vi "筛选XML解决方案.vi"(8 "error in (no error)":errorcluster caption="错误输入（无错误）", 11 "筛选输入":cluster{"platform_alarm_code":string}={"platform_alarm_code"="010002013"}) -> (0 "error out":errorcluster caption="错误输出", 3 "data":T1(array[cluster]))   [LabVIEW 2016, in "Alarm interface.lvlib"]
uses:
  Alarm interface.lvlib
  <vilib>/xml/Load XML File.vi
  <vilib>/xml/Close Reference(Node).vi
  <vilib>/xml/NI_XML.lvlib
  <resource>/objmgr/DOMUserDefRef.rc
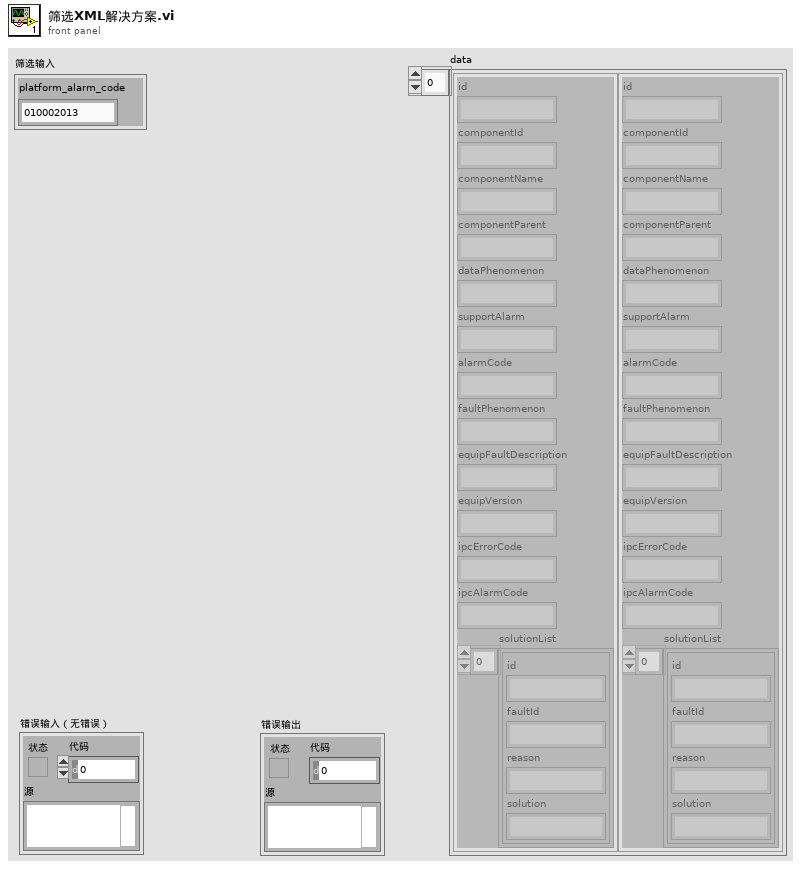
[diagram p1: front panel]
types:
  T1 = cluster{"id":string, "componentId":string, "componentName":string, "componentParent":string, "dataPhenomenon":string, "supportAlarm":string, "alarmCode":string, "faultPhenomenon":string, "equipFaultDescription":string, "equipVersion":string, "ipcErrorCode":string, "ipcAlarmCode":string, "solutionList":cluster{"id":string, "faultId":string, "reason":string, "solution":string}[]}[]
  T2 = cluster{"node text":string, "node text":string, "node text":string, "node text":string}
  T3 = cluster{"id":string, "componentId":string, "componentName":string, "componentParent":string, "dataPhenomenon":string, "supportAlarm":string, "alarmCode":string, "faultPhenomenon":string, "equipFaultDescription":string, "equipVersion":string, "ipcErrorCode":string, "ipcAlarmCode":string, "solutionList":cluster{"id":string, "faultId":string, "reason":string, "solution":string}[]}
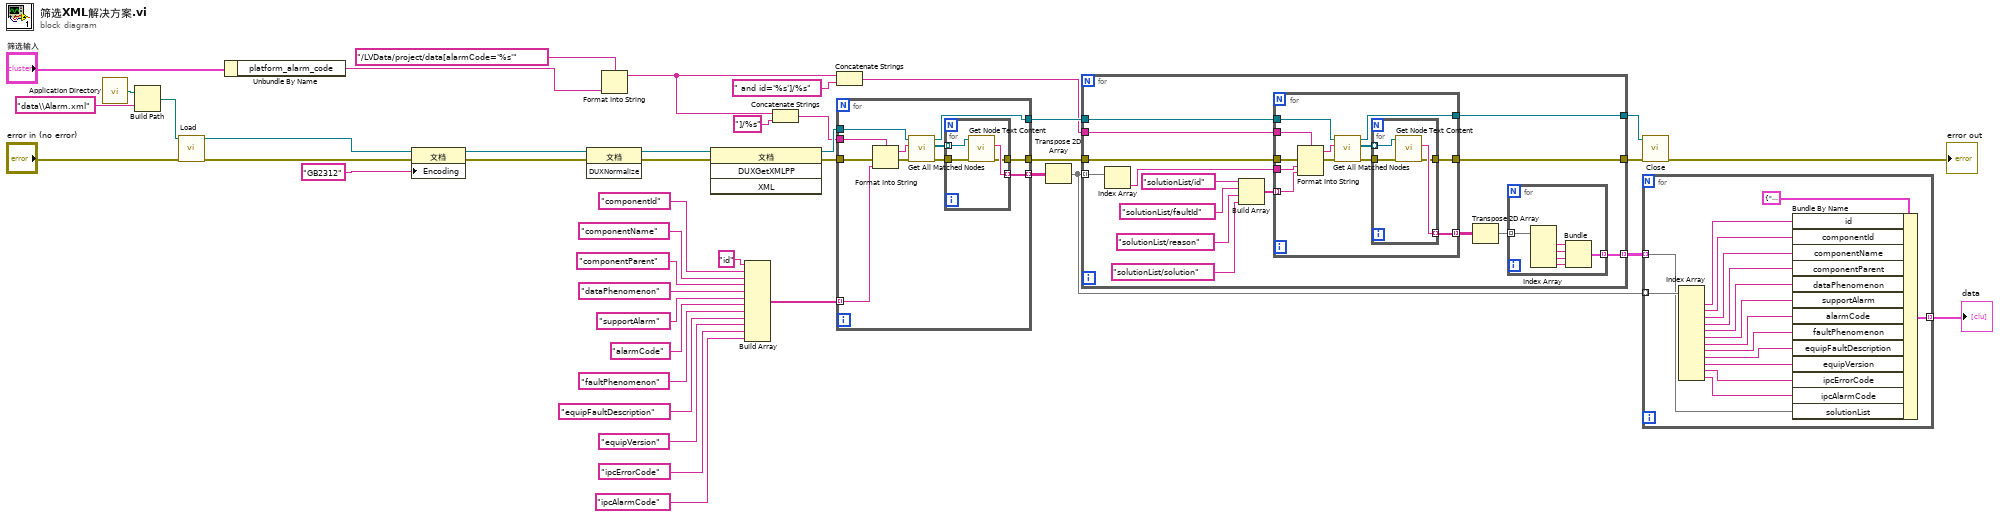
[diagram p0: block diagram]
diagram:
  n1 = call <vilib>:"Application Directory.vi"() -> ("Application Directory"=w4:path)
  n2 = Build Path(base path=w4, name or relative path="data\\Alarm.xml" ("字符串")) -> (appended path=w2:path)
  n3 = call-poly <vilib>:"Load.vi"("path to XML document"=w2, "error in (no error)"="error in (no error)") -> ("DOM document out"=w40:refnum<k20>, "error out"=w39:errorcluster)  [unwired: 11 in, 1 out]
  n4 = Unbundle By Name("筛选输入") -> ("platform_alarm_code"=w5:string)
  n5 = property on="属性节点" class="文档"(reference=w40, error in=w39, "Encoding"="GB2312" ("文档编码")) -> (reference out=w42:refnum<k20>, error out=w41:errorcluster)
  n6 = invoke on="调用节点" class="文档" method="DUXNormalize"(reference=w42, error in=w41) -> (reference out=w38:refnum<k20>, error out=w37:errorcluster)  [unwired: 1 in, 1 out]
  n7 = Format Into String(format string="/LVData/project/data[alarmCode='%s'" ("字符串"), w5) -> (resulting string=w14:string)  [unwired: 2 in, 1 out]
  n8 = invoke on="调用节点" class="文档" method="DUXGetXMLPP"(reference=w38, error in=w37) -> (reference out=w24:refnum<k20>, error out=w9:errorcluster)  [unwired: 2 in, 2 out]
  n9 = Build Array("id", "componentId", "componentName", "componentParent", "dataPhenomenon", "supportAlarm", "alarmCode", "faultPhenomenon", "equipFaultDescription", "equipVersion", "ipcErrorCode", "ipcAlarmCode") -> (w23:string[])
  n10 = Concatenate Strings(w14, "]/%s" ("字符串")) -> (w15:string)
  n11 = Concatenate Strings(w14, " and id='%s']/%s" ("字符串")) -> (w12:string)
  n12 = for {
    tunnel: w24 -> [w54]
    tunnel: w15 -> [w53]
    tunnel: w23 -> [w51] mode=indexing
    tunnel: [w49] -> w22 mode=indexing
    tunnel: [w48] -> w21
    tunnel: [w45] -> w10
    tunnel: w9 -> [w44]
    n13 = Format Into String(format string=w53, error in=w44, w51) -> (resulting string=w52:string, error out=w47:errorcluster)  [unwired: 1 in]
    n14 = call <vilib>:"Get All Matched Nodes.vi"("error in (no error)"=w47, "XPath expression"=w52, "node in"=w54) -> ("error out"=w46:errorcluster, "node result array"=w50:refnum<k20>[], "node out"=w48:refnum<k20>)  [unwired: 6 in]
    n15 = for {
      tunnel: w50 -> [w58] mode=indexing
      tunnel: [w57] -> w49 mode=indexing
      tunnel: w46 -> [w56]
      tunnel: [w55] -> w45
      n16 = call <vilib>:"Get Node Text Content.vi"("error in (no error)"=w56, "node in"=w58) -> ("error out"=w55:errorcluster, "node text"=w57:string)  [unwired: 7 in, 1 out]
    }
  }
  n17 = Transpose 2D Array(2D array=w22) -> (transposed array=w18:string[][])
  n18 = for {
    tunnel: w18 -> [w73] mode=indexing
    tunnel: w12 -> [w72]
    tunnel: w21 -> [w70]
    tunnel: [w63] -> w20
    tunnel: [w61] -> w19 mode=indexing
    tunnel: w10 -> [w60]
    tunnel: [w59] -> w8
    n19 = Index Array(array=w73) -> (element=w71:string)  [unwired: 1 in]
    n20 = Build Array("solutionList/id" ("XPath expression"), "solutionList/faultId" ("XPath expression"), "solutionList/reason" ("XPath expression"), "solutionList/solution" ("XPath expression")) -> (w65:string[])
    n21 = for {
      tunnel: w72 -> [w91]
      tunnel: w71 -> [w90]
      tunnel: w65 -> [w89] mode=indexing
      tunnel: w70 -> [w87]
      tunnel: [w85] -> w64 mode=indexing
      tunnel: [w84] -> w63
      tunnel: w60 -> [w83]
      tunnel: [w80] -> w59
      n22 = Format Into String(format string=w91, error in=w83, w90, w89) -> (resulting string=w86:string, error out=w82:errorcluster)  [unwired: 1 in]
      n23 = call <vilib>:"Get All Matched Nodes.vi"("error in (no error)"=w82, "XPath expression"=w86, "node in"=w87) -> ("error out"=w81:errorcluster, "node result array"=w88:refnum<k20>[], "node out"=w84:refnum<k20>)  [unwired: 6 in]
      n24 = for {
        tunnel: w88 -> [w95] mode=indexing
        tunnel: [w94] -> w85 mode=indexing
        tunnel: w81 -> [w93]
        tunnel: [w92] -> w80
        n25 = call <vilib>:"Get Node Text Content.vi"("error in (no error)"=w93, "node in"=w95) -> ("error out"=w92:errorcluster, "node text"=w94:string)  [unwired: 7 in, 1 out]
      }
    }
    n26 = Transpose 2D Array(2D array=w64) -> (transposed array=w62:string[][])
    n27 = for {
      tunnel: w62 -> [w79] mode=indexing
      tunnel: [w74] -> w61 mode=indexing
      n28 = Index Array(array=w79) -> (element #1=w78:string, element #2=w77:string, element #3=w76:string, element #4=w75:string)  [unwired: 4 in]
      n29 = Bundle("node text"=w78, "node text"=w77, "node text"=w76, "node text"=w75) -> (w74:T2)  [unwired: 1 in]
    }
  }
  n30 = call-poly <vilib>:"Close.vi"("error in (no error)"=w8, "node"=w20) -> ("error out"=→"error out":errorcluster)  [unwired: 7 out]
  n31 = for {
    tunnel: w18 -> [w97] mode=indexing
    tunnel: [w98] -> w17 mode=indexing
    tunnel: w19 -> [w96] mode=indexing
    n32 = Index Array(array=w97) -> (element #1=w110:string, element #2=w109:string, element #3=w108:string, element #4=w107:string, element #5=w106:string, element #6=w105:string, element #7=w104:string, element #8=w103:string, element #9=w102:string, element #10=w101:string, element #11=w100:string, element #12=w99:string)  [unwired: 12 in]
    n33 = Bundle By Name(cluster=T3 {"id"="", "componentId"="", "componentName"="", "componentParent"="", "dataPhenomenon"="", "supportAlarm"="", "alarmCode"="", "faultPhenomenon"="", "equipFaultDescription"="", "equipVersion"="", "ipcErrorCode"="", "ipcAlarmCode"="", "solutionList"=[]} ("data"), "id"=w110, "componentId"=w109, "componentName"=w108, "componentParent"=w107, "dataPhenomenon"=w106, "supportAlarm"=w105, "alarmCode"=w104, "faultPhenomenon"=w103, "equipFaultDescription"=w102, "equipVersion"=w101, "ipcErrorCode"=w100, "ipcAlarmCode"=w99, "solutionList"=w96) -> (w98:T3)
  }
  "data" <- w17
